vi "M05 Hydraulics.vi"(11 "NXT/EV3":T1) -> ()   [LabVIEW 2015]
uses:
  <vilib>/NXT/LegoClasses/BrickReference/BrickReference.lvclass
  <vilib>/NXT/Subs/LVHSConnector.ctl
  <vilib>/NXT/NXTIO Xnodes/NXTIOXNode/NXTIO.xnode
  <vilib>/NXT/NXTIO Xnodes/AddressXNode/NXTIOAddress.xnode
  <vilib>/NXT/Block Support/NXT_OutputPort.ctl
  <vilib>/NXT/NXTIO Xnodes/NXTIONodeSubVIs/LEGOResetMotors.vi
  <vilib>/NXT/NXTIO Xnodes/NXTIONodeSubVIs/NXTMotorRunDistance.vi
  <vilib>/NXT/Block Support/NXT_InputPort.ctl
  <vilib>/NXT/Dual Mode Library/Waits/Wait_Num.vi
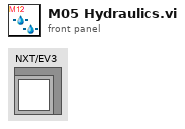
[diagram p1: front panel]
types:
  T1 = typedef "LVHSConnector.ctl" = refnum<class "BrickReference.lvclass">
  T2 = typedef "NXT_InputPort.ctl" = u32
  T3 = typedef "NXT_OutputPort.ctl" = u8
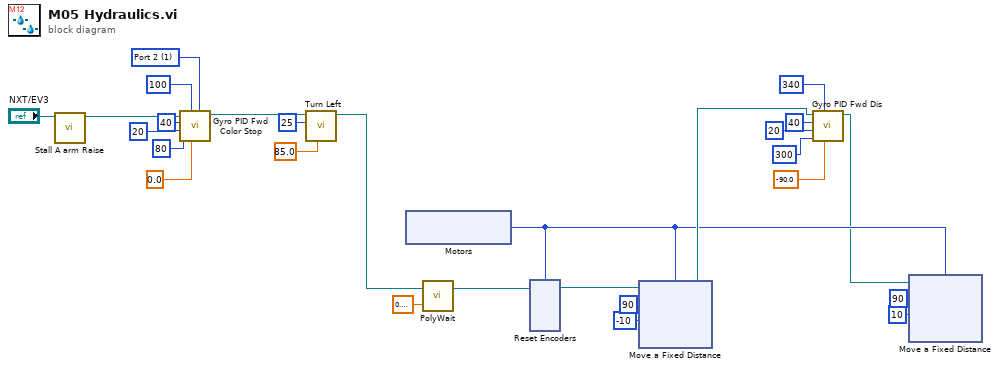
[diagram p0: block diagram]
diagram:
  w13 = T2 1 items=["Port 1", "Port 2", "Port 3", "Port 4"] ("Port")
  n1 = call "Stall A arm Raise.vi"("NXT/EV3"="NXT/EV3") -> ("NXT/EV3"=w14:T1)  [unwired: 10 in]
  n2 = call "Gyro PID Fwd Color Stop.vi"("Port"=w13, "Target angle"=sgl 0.0, "Threshold to Color"=100, "Threshold to slow"=80, "Min. speed"=20, "Max. speed"=40, "EV3 in"=w14) -> ("EV3 out"=w7:T1)  [unwired: 4 in]
  n3 = call "Turn Left.vi"("Turning angle"=sgl 85.0, "Motor B (right)"=i8 25, "EV3 in"=w7) -> ("EV3 out"=w6:T1)  [unwired: 8 in]
  n4 = xnode "Motors"() -> ("Motor"=w2:T3)
  n5 = call-poly <vilib>:"PolyWait.vi"("Time (1 sec)"=sgl 0.3, "NXT/EV3"=w6) -> ("NXT/EV3"=w25:T1)  [unwired: 2 in]
  n6 = xnode "Reset Encoders"("Motors"=w2, "NXT/EV3"=w25) -> ("NXT/EV3"=w24:T1)
  n7 = xnode "Move a Fixed Distance"("Speed 1"=i8 -10, "Distance 1"=90, "Motors"=w2, "NXT/EV3"=w24) -> ("NXT/EV3"=w5:T1)
  n8 = call "Gyro PID Fwd Dis.vi"("Target angle"=sgl -90.0, "Threshold to stop"=340, "Threshold to slow"=300, "Min. speed"=20, "Max. speed"=40, "EV3 in"=w5) -> ("EV3 out"=w1:T1)  [unwired: 5 in]
  n9 = xnode "Move a Fixed Distance"("Speed 1"=i8 10, "Distance 1"=90, "Motors"=w2, "NXT/EV3"=w1) -> ()  [unwired: 1 out]
